vi "Last_Build.vi"(0 "Current Build":string, 7 "Webpage Source":string) -> (4 "Next Build":string)   [LabVIEW 2023]
uses:
  <vilib>/regexp/Match Regular Expression.xnode
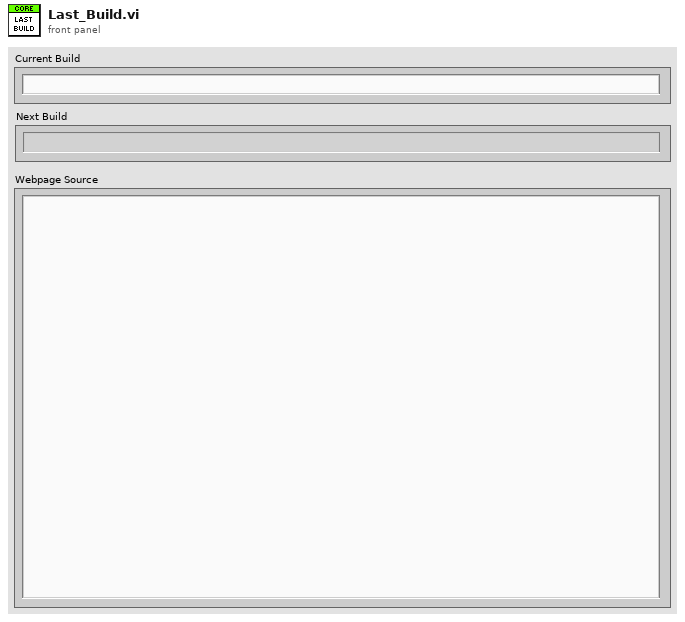
[diagram p1: front panel]
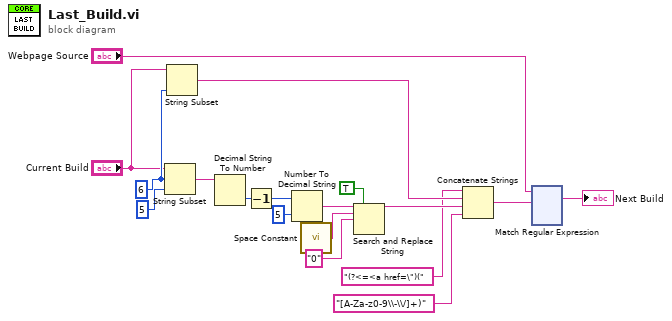
[diagram p0: block diagram]
diagram:
  w13 = 6 ("offset (0)")
  n1 = String Subset(string="Current Build", offset (0)=w13, length (rest)=5 ("length (rest)")) -> (substring=w14:string)
  n2 = String Subset(string="Current Build", length (rest)=w13) -> (substring=w12:string)  [unwired: 1 in]
  n3 = Decimal String To Number(string=w14) -> (number=w16:i32)  [unwired: 2 in, 1 out]
  n4 = Decrement(x=w16) -> (x-1=w17:i32)
  n5 = Number To Decimal String(number=w17, width (-)=i16 5) -> (decimal integer string=w10:string)
  n6 = call <vilib>:"Space Constant.vi"() -> ("String"=w9:string)
  n7 = Search and Replace String(replace all?=TRUE ("replace all? (F)"), input string=w10, search string=w9, replace string="0" ("replace string (\"\")")) -> (result string=w7:string)  [unwired: 4 in, 3 out]
  n8 = Concatenate Strings("(?<=<a href=\")(", w12, w7, "[A-Za-z0-9\\-\\/]+)") -> (w3:string)
  n9 = xnode "Match Regular Expression"("input string"="Webpage Source", "regular expression"=w3) -> ("whole match"=→"Next Build":string)  [unwired: 4 in, 4 out]
